vi "Calculator.vi"() -> ()   [LabVIEW 2016]
panel:
  out "Numeric":dbl format="%#_50f"
  in  "OK Button 15":bool
  in  "OK Button 14":bool
  in  "Button 0":bool
  in  "OK Button 12":bool
  in  "OK Button 11":bool
  in  "OK Button 10":bool
  in  "Button 9":bool
  in  "Button 8":bool
  in  "Button 7":bool
  in  "Button 6":bool
  in  "Button 5":bool
  in  "Button 4":bool
  in  "Button 3":bool
  in  "Button 2":bool
  in  "Button 1":bool
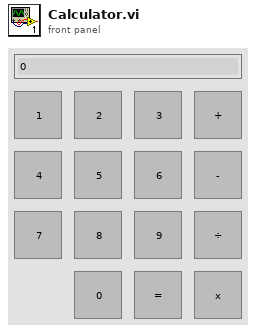
[diagram p1: front panel]
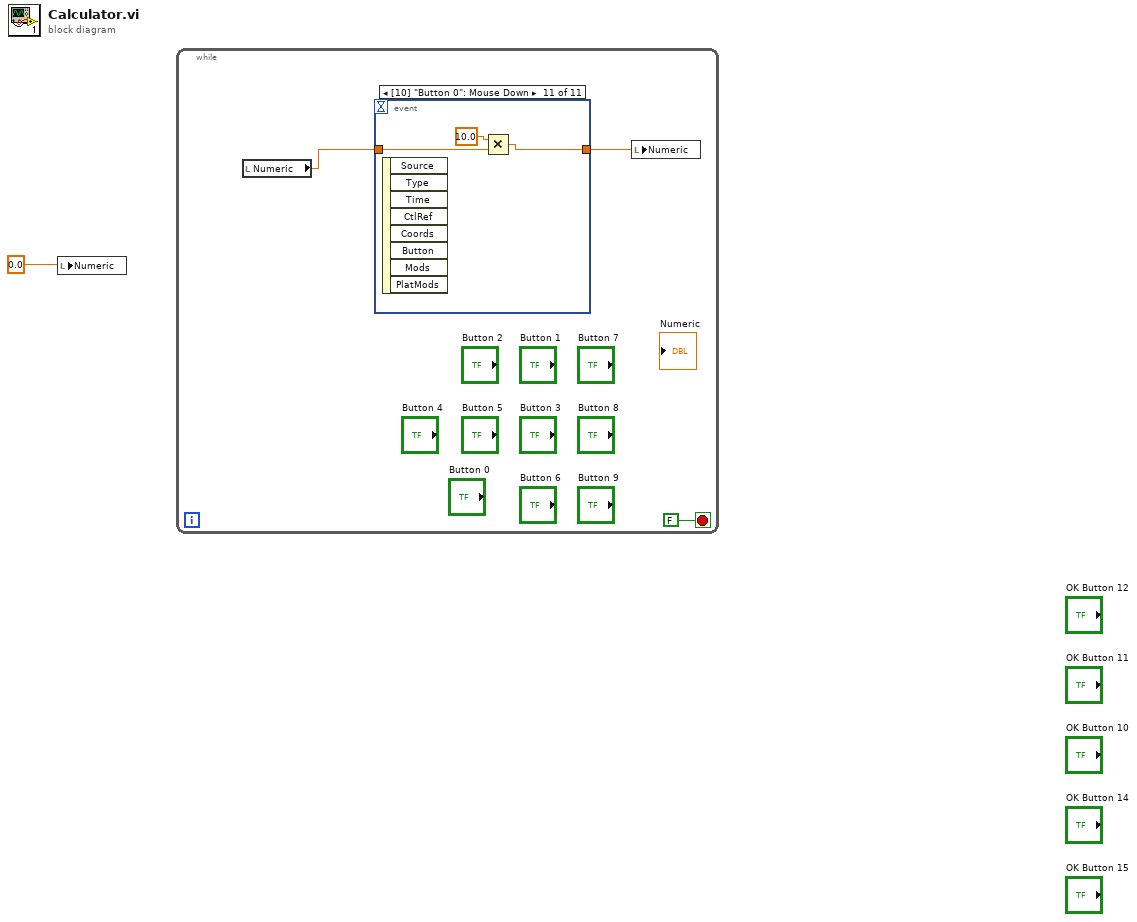
[diagram p0: block diagram]
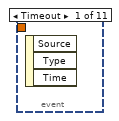
[diagram p2: hidden frame]
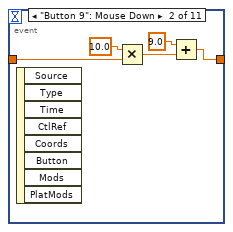
[diagram p3: hidden frame]
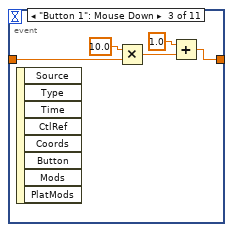
[diagram p4: hidden frame]
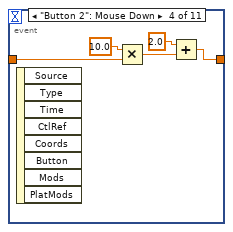
[diagram p5: hidden frame]
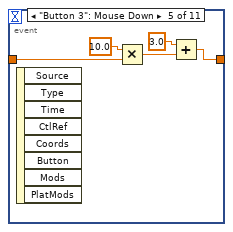
[diagram p6: hidden frame]
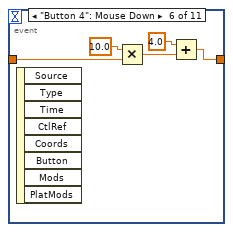
[diagram p7: hidden frame]
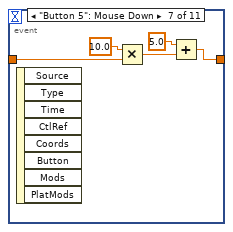
[diagram p8: hidden frame]
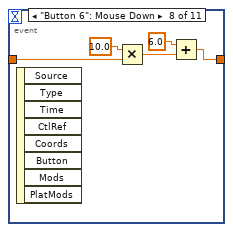
[diagram p9: hidden frame]
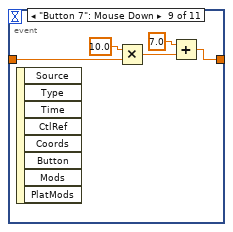
[diagram p10: hidden frame]
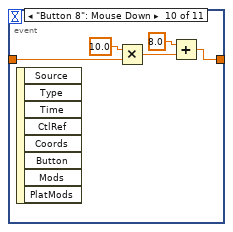
[diagram p11: hidden frame]
diagram:
  n1 = local write "Numeric"(0.0 ("Numeric")) -> ()
  n2 = while {
    stop <- FALSE stop-if-true
    n3 = local read "Numeric"() -> (w2:dbl)
    n4 = event shown="[10] \"Button 0\": Mouse Down" {
      selector: _ -> [_ _ _ _ _ _ _ _ _ _ _]
      dyn-events: _ -> [_ _ _ _ _ _ _ _ _ _ _]
      timeout: _ -> [_ _ _ _ _ _ _ _ _ _ _]
      tunnel: [_ w5 w10 w15 w20 w25 w30 w35 w40 w45 w50] -> w3
      tunnel: w2 -> [_ w9 w14 w19 w24 w29 w34 w39 w44 w49 w52]
      event Timeout {
        n5 = event-data() -> ()  [unwired: 1 in, 3 out]
      }
      event "Button 9": Mouse Down {
        n6 = event-data() -> ()  [unwired: 1 in, 8 out]
        n7 = Multiply(x=10.0 ("Numeric"), y=w9) -> (x*y=w7:dbl)
        n8 = Add(x=9.0 ("Numeric"), y=w7) -> (x+y=w5:dbl)
      }
      event "Button 1": Mouse Down {
        n9 = event-data() -> ()  [unwired: 1 in, 8 out]
        n10 = Multiply(x=10.0 ("Numeric"), y=w14) -> (x*y=w12:dbl)
        n11 = Add(x=1.0 ("Numeric"), y=w12) -> (x+y=w10:dbl)
      }
      event "Button 2": Mouse Down {
        n12 = event-data() -> ()  [unwired: 1 in, 8 out]
        n13 = Multiply(x=10.0 ("Numeric"), y=w19) -> (x*y=w17:dbl)
        n14 = Add(x=2.0 ("Numeric"), y=w17) -> (x+y=w15:dbl)
      }
      event "Button 3": Mouse Down {
        n15 = event-data() -> ()  [unwired: 1 in, 8 out]
        n16 = Multiply(x=10.0 ("Numeric"), y=w24) -> (x*y=w22:dbl)
        n17 = Add(x=3.0 ("Numeric"), y=w22) -> (x+y=w20:dbl)
      }
      event "Button 4": Mouse Down {
        n18 = event-data() -> ()  [unwired: 1 in, 8 out]
        n19 = Multiply(x=10.0 ("Numeric"), y=w29) -> (x*y=w27:dbl)
        n20 = Add(x=4.0 ("Numeric"), y=w27) -> (x+y=w25:dbl)
      }
      event "Button 5": Mouse Down {
        n21 = event-data() -> ()  [unwired: 1 in, 8 out]
        n22 = Multiply(x=10.0 ("Numeric"), y=w34) -> (x*y=w32:dbl)
        n23 = Add(x=5.0 ("Numeric"), y=w32) -> (x+y=w30:dbl)
      }
      event "Button 6": Mouse Down {
        n24 = event-data() -> ()  [unwired: 1 in, 8 out]
        n25 = Multiply(x=10.0 ("Numeric"), y=w39) -> (x*y=w37:dbl)
        n26 = Add(x=6.0 ("Numeric"), y=w37) -> (x+y=w35:dbl)
      }
      event "Button 7": Mouse Down {
        n27 = event-data() -> ()  [unwired: 1 in, 8 out]
        n28 = Multiply(x=10.0 ("Numeric"), y=w44) -> (x*y=w42:dbl)
        n29 = Add(x=7.0 ("Numeric"), y=w42) -> (x+y=w40:dbl)
      }
      event "Button 8": Mouse Down {
        n30 = event-data() -> ()  [unwired: 1 in, 8 out]
        n31 = Multiply(x=10.0 ("Numeric"), y=w49) -> (x*y=w47:dbl)
        n32 = Add(x=8.0 ("Numeric"), y=w47) -> (x+y=w45:dbl)
      }
      event "Button 0": Mouse Down {
        n33 = event-data() -> ()  [unwired: 1 in, 8 out]
        n34 = Multiply(x=10.0 ("Numeric"), y=w52) -> (x*y=w50:dbl)
      }
    }
    n35 = local write "Numeric"(w3) -> ()
  }
